vi "Save LUT to Disk.vi"(10 "file (use dialog)":path, 11 "Blaze Data":dbl[](array[numeric])) -> (3 "file (use dialog) out":path)   [LabVIEW 2020]
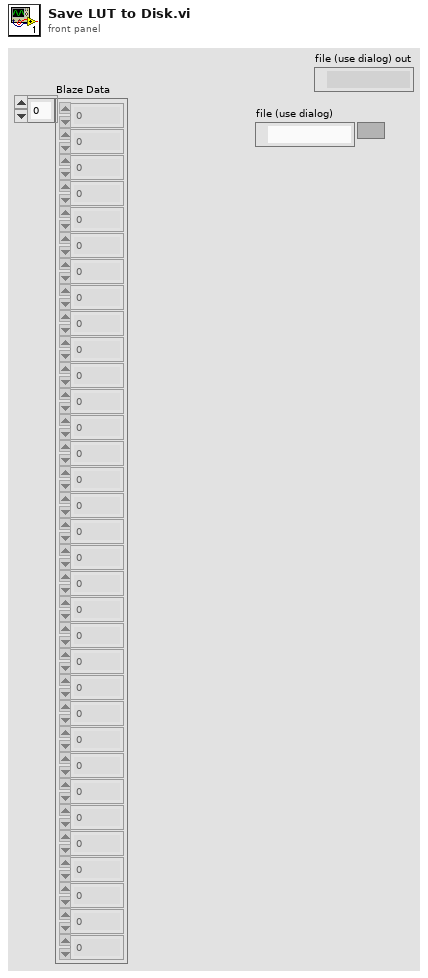
[diagram p1: front panel]
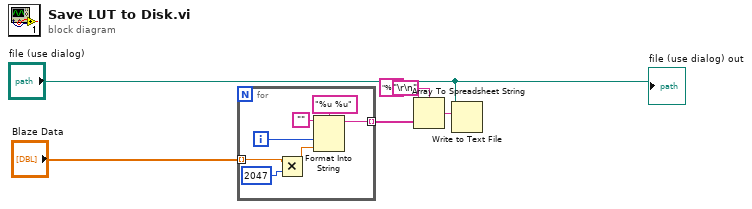
[diagram p0: block diagram]
diagram:
  n1 = for {
    tunnel: "Blaze Data" -> [w10] mode=indexing
    tunnel: [w11] -> w2 mode=indexing
    i -> [w7]
    n2 = Multiply(x=w10, y=2047) -> (x*y=w9:dbl)
    n3 = Format Into String(format string="%u %u", initial string="", w7, w9) -> (resulting string=w11:string)  [unwired: 1 in, 1 out]
  }
  n4 = Array To Spreadsheet String(delimiter (Tab)="\r\n", array=w2, 3:"%s") -> (spreadsheet string=w3:string)
  n5 = Write to Text File(file (use dialog)="file (use dialog)", text=w3) -> ()  [unwired: 2 in, 3 out]
  "file (use dialog) out" <- "file (use dialog)"
